vi "Show Error.vi"(6 "Last Error Message in":string, 8 "Error In":errorcluster, 11 "Error Message in":string) -> (0 "Error Out":errorcluster, 4 "Error Message out":string)   [LabVIEW 2019]
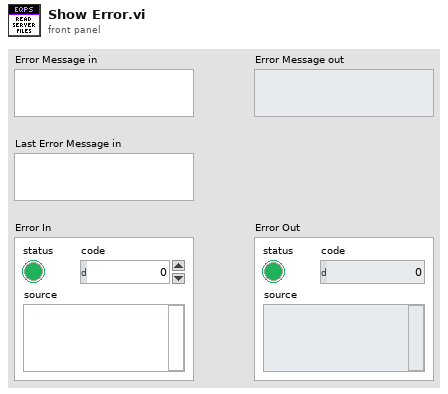
[diagram p1: front panel]
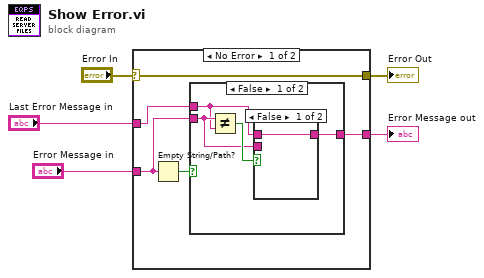
[diagram p0: block diagram]
diagram:
  n1 = case shown="No Error" "Error In" {
    selector: "Error In" -> [w7 w19]
    tunnel: [w7 w19] -> w4
    tunnel: [w9 w18] -> w3
    tunnel: "Error Message in" -> [w6 w18]
    tunnel: "Last Error Message in" -> [w8 _]
    frame No Error {
      n2 = Empty String/Path?(string/path=w6) -> (empty?=w10:bool)
      n3 = case shown="False" w10 {
        tunnel: [w11 w17] -> w9
        tunnel: w8 -> [w12 w17]
        tunnel: w6 -> [w13 _]
        frame False {
          n4 = Not Equal?(x=w13, y=w12) -> (x != y?=w14:bool)
          n5 = case shown="False" w14 {
            tunnel: w13 -> [_ w16]
            tunnel: w12 -> [w15 _]
            tunnel: [w15 w16] -> w11
            frame False {
            }
            frame True {
            }
          }
        }
        frame True {
        }
      }
    }
    frame Error {
    }
  }
  "Error Out" <- w4
  "Error Message out" <- w3
